vi "LAS-CTS_SingleSpotCurrentMonitor.vi"() -> ()   [LabVIEW 2024]
uses:
  <vilib>/httpClient/LabVIEWHTTPClient.lvlib
  <vilib>/Analysis/NI_AALBase.lvlib
panel:
  out "Waveform Graph":dbl[](graph)
  in  "Ammeter Range":dbl(ring)=0.02 items=["20 mA"=0.02, "2 mA"=0.002, "200 uA"=0.0002, "20 uA"=2e-05, "2 uA"=2e-06, "200 nA"=2e-07, "20 nA"=2e-08, "2 nA"=2e-09, "200 pA"=2e-10, "20 pA"=2e-11]
  out "last file name":string
  in  "base filename":string
  in  "file number":i32 format="%03d"
  out "# of samples":i32
  in  "Z position (mirror mm)":string
  in  "X position (mirror mm)":string
  in  "Target ID":string
  in  "data filepath":path
  in  "Number of Pulses":i32
  out "Laser On/Off":bool
  out "Pulses Remaining":i32
  out "Laser Energy (uJ)":dbl format="%#.3f"
  in  "# data points":i32
  in  "Energy Meter":refnum<visa-resource-name>
  in  "Keithly":refnum<visa-resource-name>
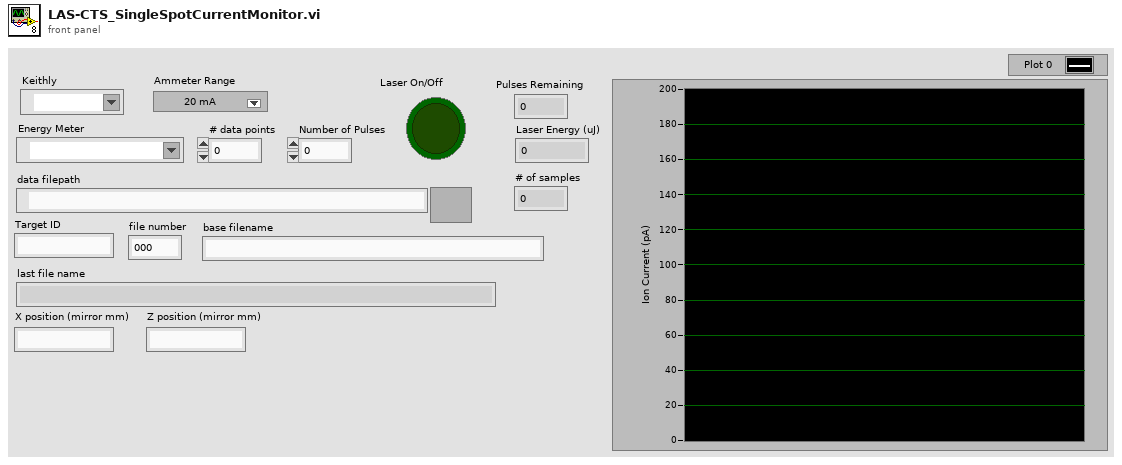
[diagram p1: front panel]
types:
  T1 = enum16{"open", "replace", "create", "open or create", "replace or create", "replace or create with confirmation"}
  T2 = typedef "LabVIEWHTTPClient.lvlib/ClientHandle.ctl" = refnum<k1>
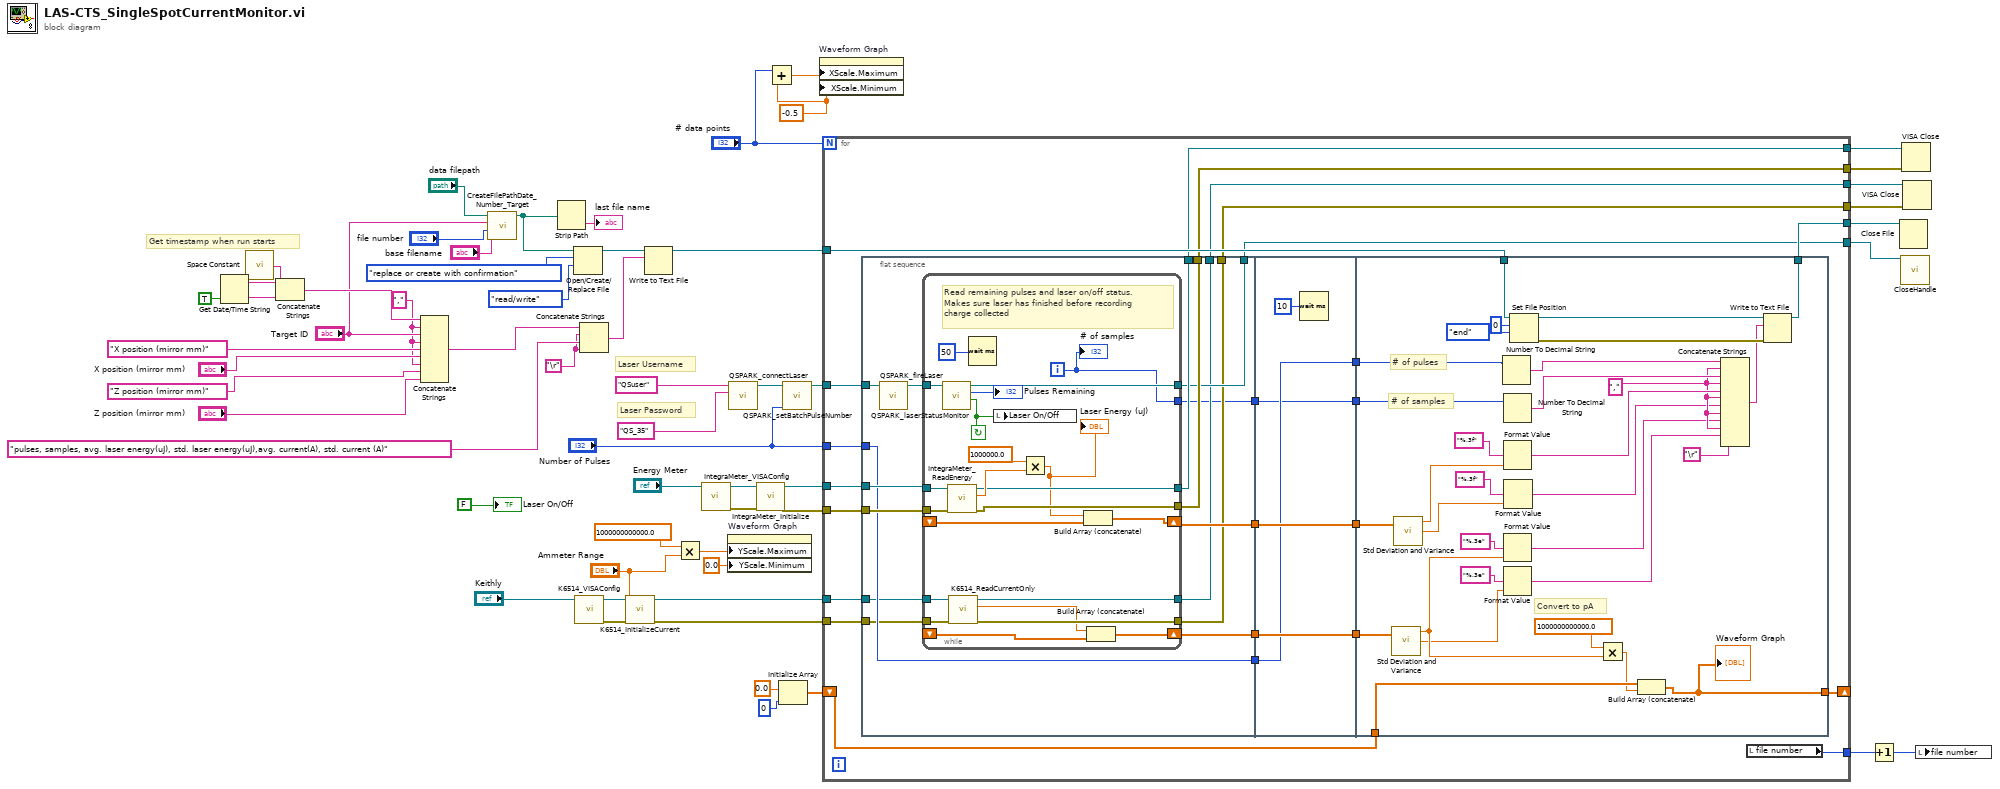
[diagram p0: block diagram]
diagram:
  w2 = -0.5 ("X Scale.Range:Minimum")
  w13 = "," ("string")
  w44 = "\r"
  # "Get timestamp when run starts"
  # "Laser Password"
  # "Laser Username"
  n1 = Get Date/Time String(want seconds? (F)=TRUE) -> (date string=w43:string, time string=w42:string)  [unwired: 2 in]
  n2 = call <vilib>:"Space Constant.vi"() -> ("String"=w41:string)
  n3 = Concatenate Strings(w43, w41, w42) -> (w39:string)
  n4 = Concatenate Strings(w39, w13, "Target ID", w13, "X position (mirror mm)" ("string"), "X position (mirror mm)", w13, "Z position (mirror mm)" ("string"), "Z position (mirror mm)") -> (w38:string)
  n5 = call "CreateFilePathDate_Number_Target.vi"("base filename"="base filename", "file number"="file number", "Target ID"="Target ID", "data filepath"="data filepath") -> ("appended path"=w25:path)  [unwired: 7 in]
  n6 = Strip Path(path=w25) -> (name=→"last file name":string)  [unwired: 1 out]
  n7 = Open/Create/Replace File(file path (use dialog)=w25, operation (0:open)=T1."replace or create with confirmation", access (0:read/write)=enum16{"read/write", "read-only", "write-only"}."read/write") -> (refnum out=w47:refnum<file>)  [unwired: 3 in, 2 out]
  n8 = call "K6514_VISAConfig.vi"("VISA resource name"="Keithly") -> ("error out"=w58:errorcluster, "reference out"=w57:refnum<visa-resource-name>)  [unwired: 9 in]
  n9 = Concatenate Strings(w38, w44, "pulses, samples, avg. laser energy(uJ), std. laser energy(uJ),avg. current(A), std. current (A)", w44) -> (w45:string)
  n10 = call "K6514_InitializeCurrent.vi"("error in (no error)"=w58, "Range"="Ammeter Range", "VISA resource name"=w57) -> ("error out"=w19:errorcluster, "VISA resource name out"=w23:refnum<visa-resource-name>)  [unwired: 7 in]
  n11 = Write to Text File(file (use dialog)=w47, text=w45) -> (refnum out=w37:refnum<file>)  [unwired: 2 in, 2 out]
  n12 = Multiply(x=1000000000000.0, y="Ammeter Range") -> (x*y=w7:dbl)
  n13 = call "IntegraMeter_VISAConfig.vi"("VISA resource name"="Energy Meter") -> ("error out"=w8:errorcluster, "reference out"=w55:refnum<visa-resource-name>)  [unwired: 9 in]
  n14 = property on="Waveform Graph" class="WFGraph (strict)"("YScale.Maximum"=w7, "YScale.Minimum"=0.0 ("Y Scale.Range:Minimum")) -> ()  [unwired: 2 in, 2 out]
  n15 = call "QSPARK_connectLaser.vi"("password"="QS_35", "username"="QSuser") -> ("client handle out"=w22:T2)  [unwired: 9 in]
  n16 = call "IntegraMeter_Initialize.vi"("error in"=w8, "VISA resource name"=w55) -> ("error out"=w52:errorcluster, "VISA resource name out"=w53:refnum<visa-resource-name>)  [unwired: 8 in]
  n17 = Add(x="# data points", y=w2) -> (x+y=w3:dbl)
  n18 = Initialize Array(0.0 ("element"), 0 ("dimension size")) -> (w9:dbl[])
  n19 = call "QSPARK_setBatchPulseNumber.vi"("Number of Pulses"="Number of Pulses", "client handle"=w22) -> ("client handle out"=w51:T2)  [unwired: 9 in]
  n20 = property on="Waveform Graph" class="WFGraph (strict)"("XScale.Maximum"=w3, "XScale.Minimum"=w2) -> ()  [unwired: 2 in, 2 out]
  n21 = for {
    N: "# data points" -> [_]
    tunnel: w53 -> [w82]
    tunnel: w52 -> [w81]
    tunnel: w51 -> [w80]
    tunnel: w37 -> [w79]
    tunnel: [w78] -> w36
    tunnel: [w77] -> w35
    tunnel: [w76] -> w34
    tunnel: [w75] -> w33
    tunnel: "Number of Pulses" -> [w73]
    tunnel: [w70] -> w26
    tunnel: w23 -> [w69]
    tunnel: w19 -> [w68]
    tunnel: [w67] -> w18
    tunnel: [w66] -> w17
    shift-right: [w59] -> _
    shift-left: w9 -> [w60]
    n22 = flat-sequence {
      tunnel: w82 -> [w97]
      tunnel: w81 -> [w96]
      tunnel: w80 -> [w94]
      tunnel: [w93] -> w78
      tunnel: [w92] -> w77
      tunnel: [w91] -> w75
      tunnel: [w90] -> w74
      tunnel: w73 -> [w90]
      tunnel: [w89] -> w72
      tunnel: w69 -> [w88]
      tunnel: w68 -> [w87]
      tunnel: [w86] -> w67
      tunnel: [w85] -> w66
      tunnel: [w84] -> w64
      tunnel: [w83] -> w61
      tunnel: w74 -> [w121]
      tunnel: w72 -> [w123]
      tunnel: [w123] -> w71
      tunnel: [w122] -> w65
      tunnel: w64 -> [w122]
      tunnel: [w121] -> w63
      tunnel: [w120] -> w62
      tunnel: w61 -> [w120]
      tunnel: w79 -> [w147]
      tunnel: [w146] -> w76
      tunnel: w71 -> [w144]
      tunnel: w65 -> [w140]
      tunnel: w63 -> [w130]
      tunnel: w62 -> [w129]
      tunnel: w60 -> [w127]
      tunnel: [w125] -> w59
      frame #0 {
        n23 = call "QSPARK_fireLaser.vi"("client handle"=w94) -> ("client handle out"=w95:T2)  [unwired: 10 in]
        n24 = while {
          tunnel: w95 -> [w118]
          tunnel: [w117] -> w91
          shift-right: [w111] -> w89
          shift-left: _ -> [w114]
          tunnel: w97 -> [w110]
          tunnel: w96 -> [w109]
          tunnel: [w108] -> w93
          tunnel: [w107] -> w92
          tunnel: w88 -> [w105]
          tunnel: w87 -> [w104]
          shift-right: [w103] -> w84
          shift-left: _ -> [w102]
          tunnel: [w101] -> w86
          tunnel: [w100] -> w85
          tunnel: [w98] -> w83
          i -> [w98]
          stop <- w115 continue-if-true
          # "Read remaining pulses and laser on/off status. \nMakes sure laser has finished before recording \ncharge collected"
          n25 = call "QSPARK_laserStatusMonitor.vi"("client handle"=w118) -> ("laser on?"=w115:bool, "remaining pulses"=→"Pulses Remaining":i32, "client handle out"=w117:T2)  [unwired: 8 in]
          n26 = call "IntegraMeter_ReadEnergy.vi"("error in (no error)"=w109, "VISA resource name"=w110) -> ("error out"=w107:errorcluster, "Laser Energy (J)"=w112:dbl, "VISA resource name out"=w108:refnum<visa-resource-name>)  [unwired: 7 in]
          n27 = call "K6514_ReadCurrentOnly.vi"("error in (no error)"=w104, "VISA resource name"=w105) -> ("error out"=w100:errorcluster, "Current (A)"=w99:dbl, "VISA resource name out"=w101:refnum<visa-resource-name>)  [unwired: 5 in, 1 out]
          n28 = Wait (ms)(milliseconds to wait=u32 50 ("millisecond multiple")) -> ()  [unwired: 1 out]
          n29 = local write "Laser On/Off"(w115) -> ()
          n30 = Multiply(x=1000000.0, y=w112) -> (x*y=w106:dbl)
          "Laser Energy (uJ)" <- w106
          n31 = Build Array (concatenate)(w106, w114) -> (w111:dbl[])
          n32 = Build Array (concatenate)(w99, w102) -> (w103:dbl[])
          "# of samples" <- w98
        }
      }
      frame #1 {
        n33 = Wait (ms)(milliseconds to wait=u32 10) -> ()  [unwired: 1 out]
      }
      frame #2 {
        w135 = "," ("string")
        # "# of samples"
        # "# of pulses"
        # "Convert to pA"
        n34 = call <vilib>:"Std Deviation and Variance.vi"("X"=w140) -> ("mean"=w142:dbl, "standard deviation"=w136:dbl)  [unwired: 1 in, 1 out]
        n35 = call <vilib>:"Std Deviation and Variance.vi"("X"=w144) -> ("mean"=w143:dbl, "standard deviation"=w138:dbl)  [unwired: 1 in, 1 out]
        n36 = Number To Decimal String(number=w130) -> (decimal integer string=w131:string)  [unwired: 1 in]
        n37 = Number To Decimal String(number=w129) -> (decimal integer string=w150:string)  [unwired: 1 in]
        n38 = Format Value(format string="%.3f", value (0)=w143) -> (output string=w148:string)  [unwired: 1 in]
        n39 = Format Value(format string="%.3e", value (0)=w142) -> (output string=w133:string)  [unwired: 1 in]
        n40 = Format Value(format string="%.3e", value (0)=w136) -> (output string=w132:string)  [unwired: 1 in]
        n41 = Format Value(format string="%.3f", value (0)=w138) -> (output string=w134:string)  [unwired: 1 in]
        n42 = Set File Position(offset (in bytes) (0)=i64 0, refnum=w147, from (0:start)=enum16{"start", "end", "current"}."end") -> (refnum out=w152:refnum<file>, error out=w155:errorcluster)  [unwired: 1 in]
        n43 = Multiply(x=1000000000000.0, y=w142) -> (x*y=w126:dbl)
        n44 = Build Array (concatenate)(w127, w126) -> (w125:dbl[])
        "Waveform Graph" <- w125
        n45 = Concatenate Strings(w131, w135, w150, w135, w148, w135, w134, w135, w133, w135, w132, "\r") -> (w151:string)
        n46 = Write to Text File(file (use dialog)=w152, text=w151, error in=w155) -> (refnum out=w146:refnum<file>)  [unwired: 1 in, 2 out]
      }
    }
    n47 = local read "file number"() -> (w70:i32)
  }
  n48 = Increment(x=w26) -> (x+1=w27:i32)
  n49 = Close File(refnum=w34) -> ()  [unwired: 1 in, 2 out]
  n50 = call <vilib>:"CloseHandle.vi"("client handle"=w33) -> ()  [unwired: 14 in, 1 out]
  n51 = VISA Close(VISA resource name=w36, error in (no error)=w35) -> ()  [unwired: 1 out]
  n52 = VISA Close(VISA resource name=w18, error in (no error)=w17) -> ()  [unwired: 1 out]
  n53 = local write "file number"(w27) -> ()
  "Laser On/Off" <- FALSE ("Laser On/Off")
